vi "String-Based Queued State Machine_ACBMOD.vi"() -> ()   [LabVIEW 2015]
panel:
  in  "OK":bool
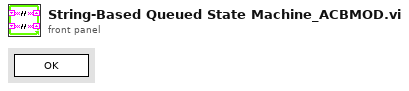
[diagram p1: front panel]
types:
  T1 = enum32{"Invalid", "Standard", "Closed", "Hidden", "Minimized", "Maximized"}
  T2 = enum32{"invalid app kind", "Development System", "Run Time System", "Student Edition", "Embedded LabVIEW", "Evaluation", "Custom"}
  T3 = cluster{"Core":cluster{"Current VI Reference":refnum<vi>, "Close Panel on Exit?":bool}, "Your Boolean data":bool, "Your string data":string}
  T4 = cluster{"Current VI Reference":refnum<vi>, "Close Panel on Exit?":bool}
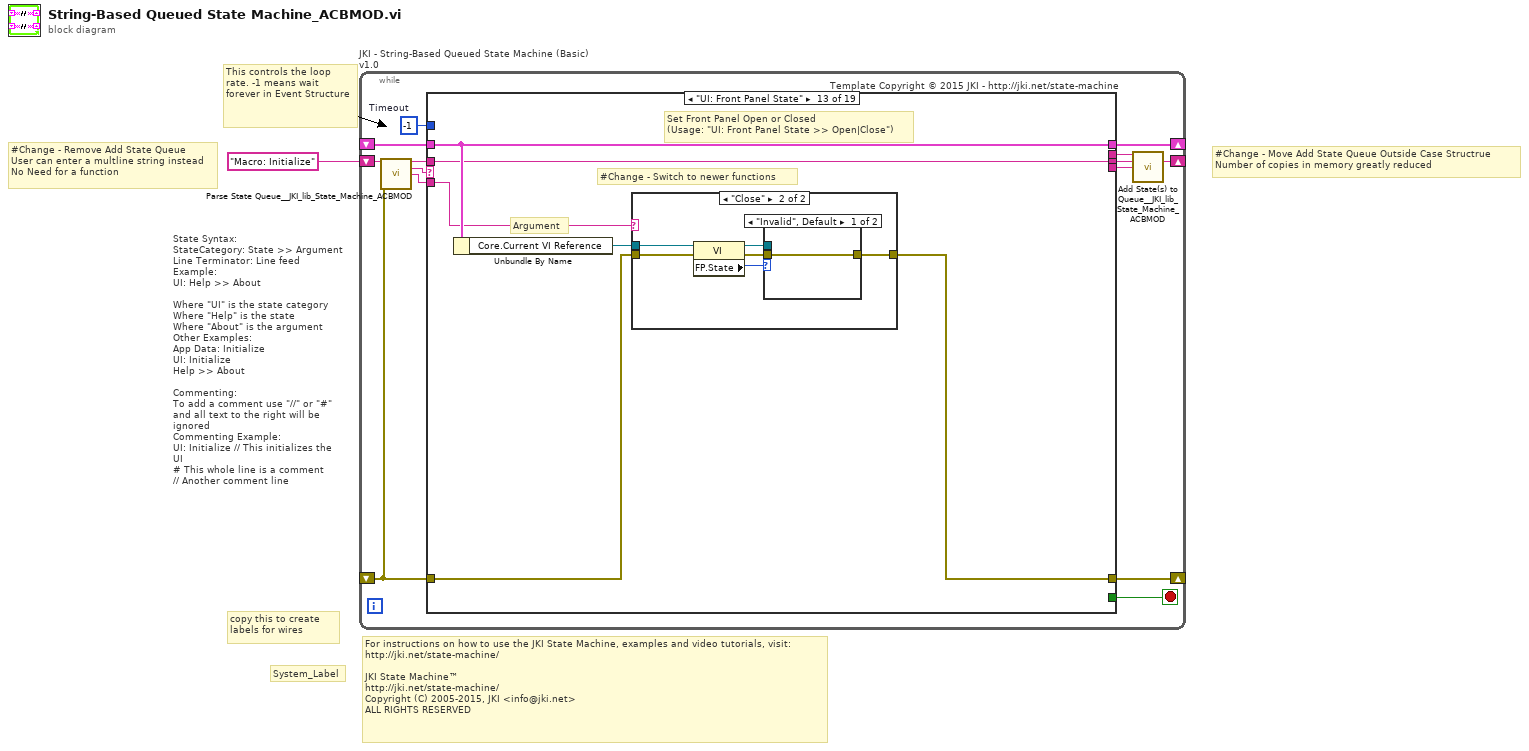
[diagram p0: block diagram]
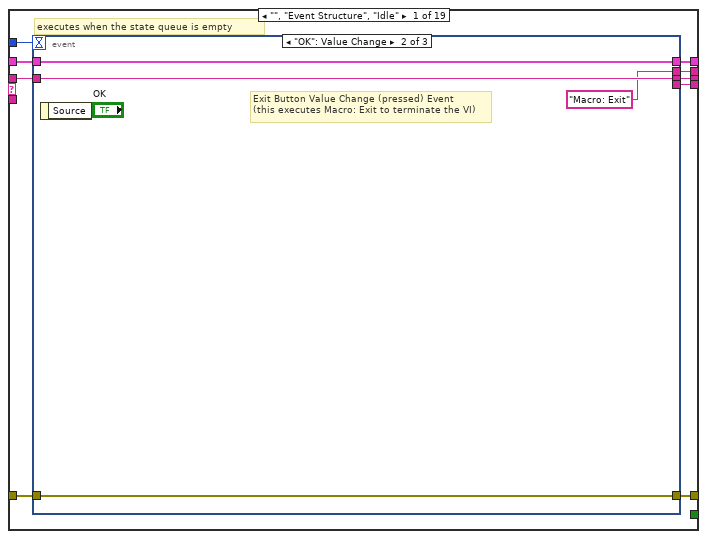
[diagram p2: hidden frame]
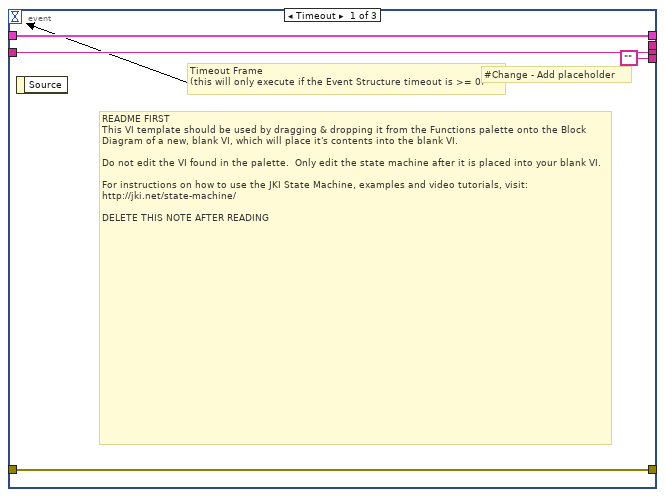
[diagram p3: hidden frame]
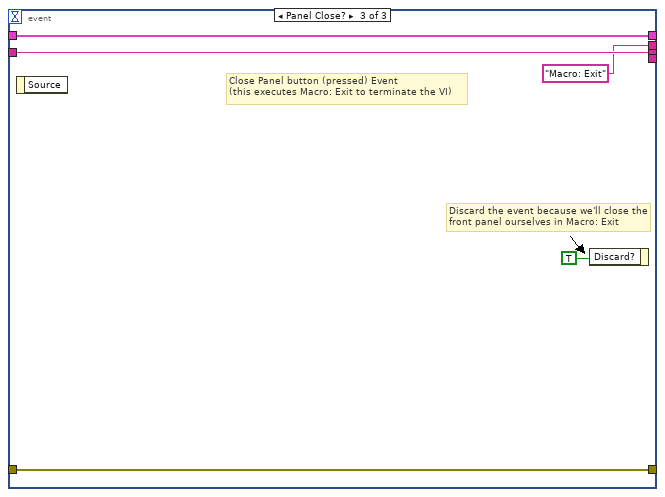
[diagram p4: hidden frame]
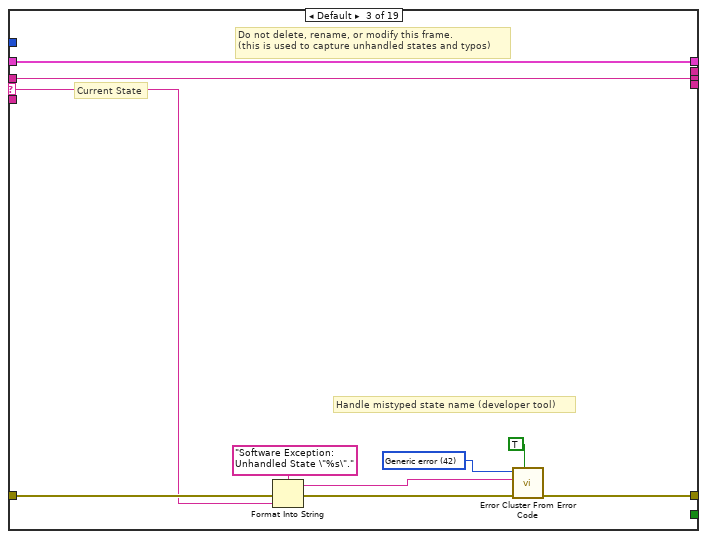
[diagram p6: hidden frame]
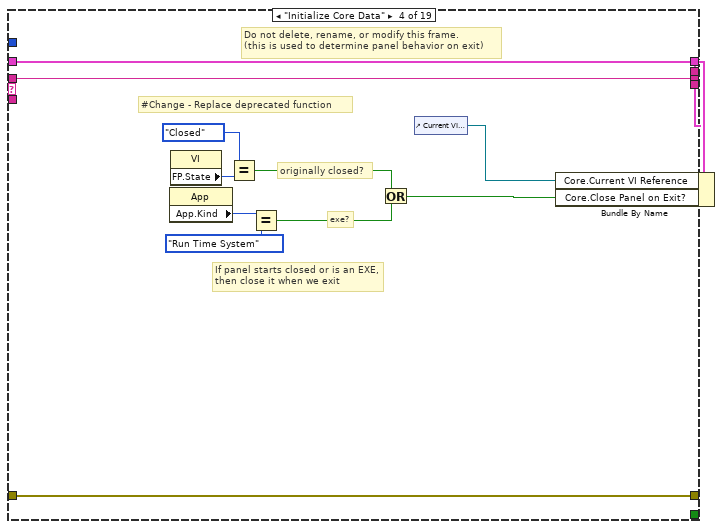
[diagram p7: hidden frame]
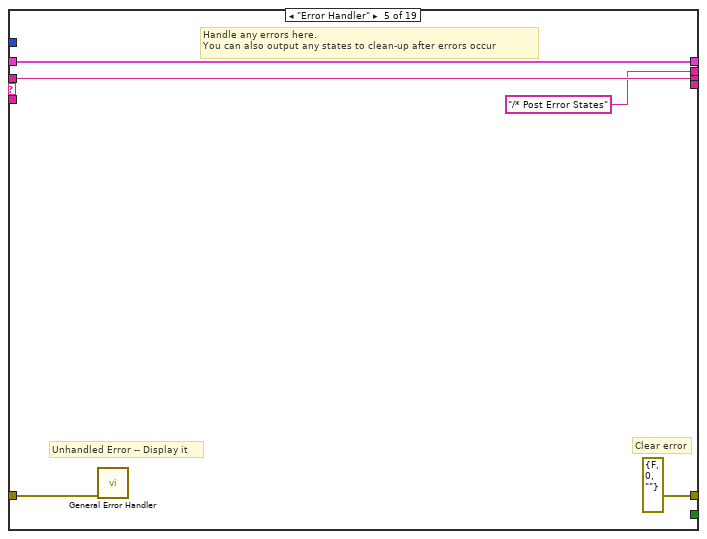
[diagram p8: hidden frame]
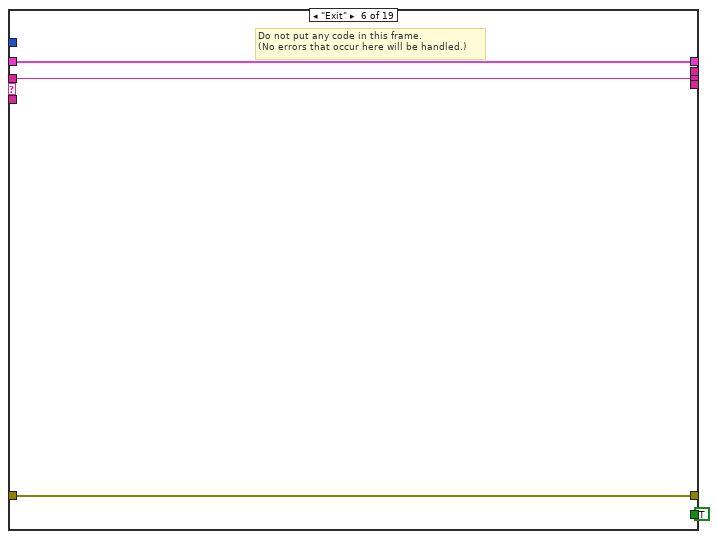
[diagram p9: hidden frame]
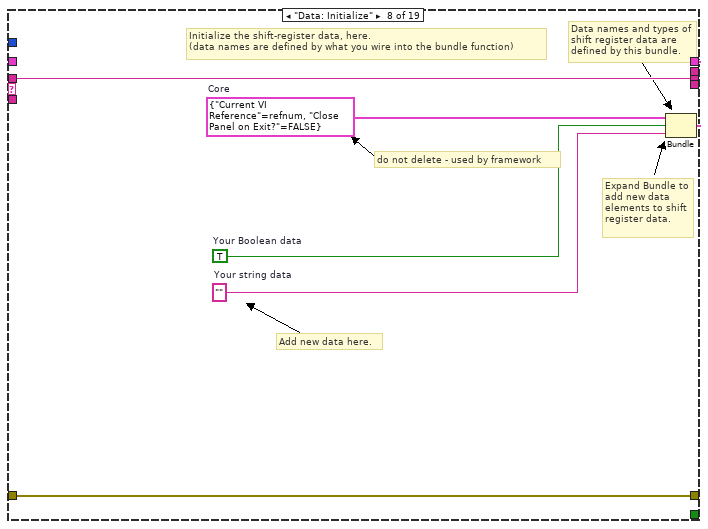
[diagram p11: hidden frame]
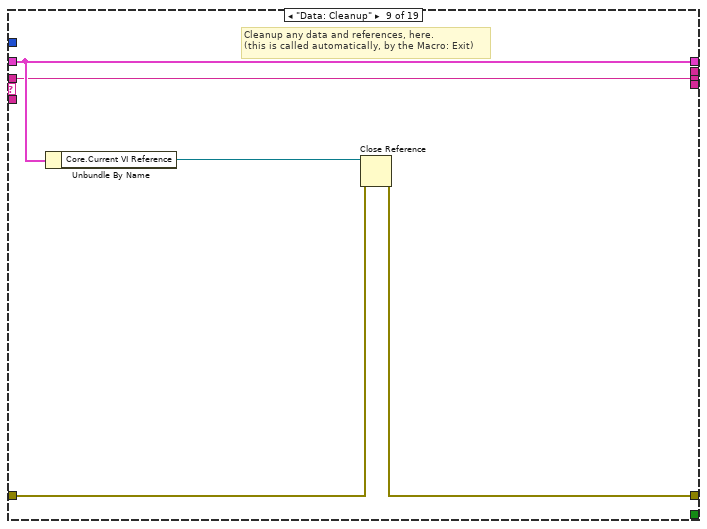
[diagram p12: hidden frame]
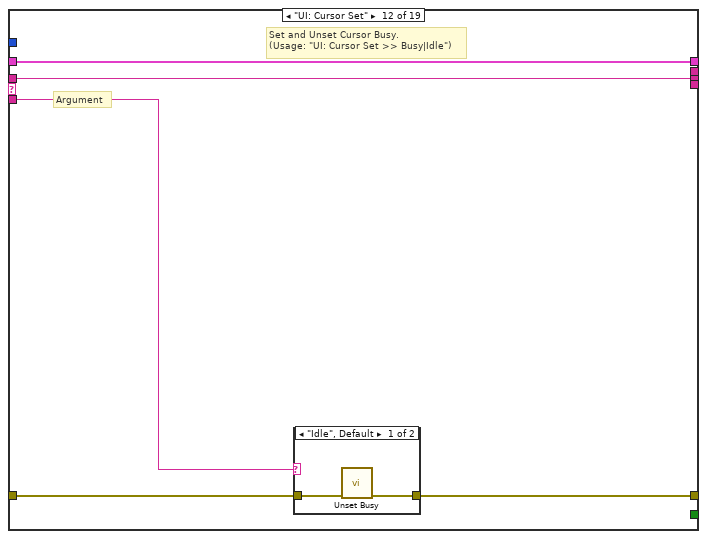
[diagram p15: hidden frame]
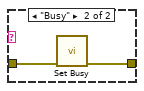
[diagram p16: hidden frame]
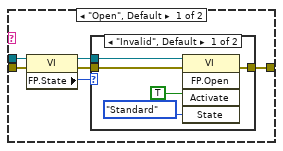
[diagram p17: hidden frame]
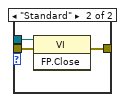
[diagram p19: hidden frame]
diagram:
  # "#Change - Move Add State Queue Outside Case Structrue\nNumber of copies in memory greatly reduced"
  # "#Change - Remove Add State Queue\nUser can enter a multline string instead\nNo Need for a function"
  # "For instructions on how to use the JKI State Machine, examples and video tutorials, visit:\nhttp://jki.net/state-machine/\n\nJKI State Machine™\nhttp://jki.net/state-machine/\nCopyright (C) 2005-2015, JKI <info@jki.net>\nALL RIGHTS RESERVED"
  # "State Syntax:\nStateCategory: State >> Argument\nLine Terminator: Line feed\nExample:\nUI: Help >> About\n\nWhere \"UI\" is the state category\nWhere \"Help\" is the state\nWhere \"About\" is the argument\nOther Examples:\nApp Data: Initialize\nUI: Initialize\nHelp >> About\n\nCommenting:\nTo add a comment use \"//\" or \"#\" and all text to the right will be ignored\nCommenting Example:\nUI: Initialize // This initializes the UI\n# This whole line is a comment\n// Another comment line"
  # "copy this to create labels for wires"
  # "This controls the loop rate. -1 means wait forever in Event Structure"
  # "System_Label"
  n1 = while "JKI - String-Based Queued State Machine (Basic) v1.0" {
    shift-right: [w9] -> _
    shift-left: _ -> [w8]
    shift-right: [w11] -> _
    shift-left: _ -> [w6]
    shift-right: [w4] -> _
    shift-left: "Macro: Initialize" -> [w12]
    stop <- w10 stop-if-true
    w7 = -1  # Timeout
    # "Template Copyright © 2015 JKI - http://jki.net/state-machine"
    n2 = call "Parse State Queue__JKI_lib_State_Machine_ACBMOD.vi"("State Queue"=w12, "Error In"=w6) -> ("Remaining States"=w14:string, "Current State"=w15:string, "Arguments"=w13:string)  [unwired: 11 in]
    n3 = case shown="\"UI: Front Panel State\"" w15 {
      selector: w15 -> [_ _ w42 _ _ _ _ _ _ _ _ _ _ _ _ _ _ _ _]
      tunnel: w14 -> [w24 w38 w41 w51 w64 w68 w72 w75 w81 w86 w89 w92 w101 w129 w133 w137 w145 w148 w151]
      tunnel: w13 -> [_ _ _ _ _ _ _ _ _ _ _ w93 w102 _ _ _ _ _ _]
      tunnel: w8 -> [w22 w39 w44 w58 w66 w71 w73 _ w82 w87 w91 w96 w104 w130 w134 w143 w146 w149 w152]
      tunnel: [w21 w40 w46 w61 errorcluster {"status"=FALSE, "code"=0, "source"=""} ("error out") w70 w74 w79 w83 w88 w90 w94 w105 w131 w135 w144 w147 w150 w153] -> w11
      tunnel: w6 -> [w20 w40 w45 w61 w65 w70 w74 w79 w84 w88 w90 w95 w106 w131 w135 w144 w147 w150 w153]
      tunnel: [w23 w38 w41 w51 w64 w68 w72 w75 w81 w86 w89 w92 w101 w129 w133 w137 w145 w148 w151] -> w5
      tunnel: [_ _ _ _ _ TRUE _ _ _ _ _ _ _ _ _ _ _ _ _] -> w10
      tunnel: [w19 w39 w44 w62 w66 w71 w73 w80 w82 w87 w91 w96 w104 w130 w134 w143 w146 w149 w152] -> w9
      tunnel: w7 -> [w18 _ _ _ _ _ _ _ _ _ _ _ _ _ _ _ _ _ _]
      tunnel: [w17 _ _ _ "/* Post Error States" _ _ _ _ _ _ _ _ _ w132 w136 _ _ _] -> w3
      tunnel: [w16 _ _ _ _ _ _ _ _ _ _ _ _ _ _ _ _ _ _] -> w2
      frame "", "Event Structure", "Idle" {
        # "executes when the state queue is empty"
        n4 = event shown="[1] \"OK\": Value Change" {
          selector: _ -> [_ _ _]
          dyn-events: _ -> [_ _ _]
          timeout: w18 -> [_ _ _]
          tunnel: w24 -> [w26 w30 w34]
          tunnel: [w26 w30 w34] -> w23
          tunnel: w22 -> [w27 w31 w36]
          tunnel: [w28 w32 w37] -> w21
          tunnel: w20 -> [w28 w32 w37]
          tunnel: [w27 w31 w36] -> w19
          tunnel: [_ "Macro: Exit" "Macro: Exit"] -> w17
          tunnel: ["" _ _] -> w16
          event Timeout {
            # "#Change - Add placeholder"
            # "README FIRST\nThis VI template should be used by dragging & dropping it from the Functions palette onto the Block Diagram of a new, blank VI, which will place it's contents into the blank VI.\n\nDo not edit the VI found in the palette.  Only edit the state machine after it is placed into your blank VI.\n\nFor instructions on how to use the JKI State Machine, examples and video tutorials, visit:\nhttp://jki.net/state-machine/\n\nDELETE THIS NOTE AFTER READING"
            # "Timeout Frame\n(this will only execute if the Event Structure timeout is >= 0)"
            n5 = event-data() -> ()  [unwired: 1 in, 1 out]
          }
          event "OK": Value Change {
            # "Exit Button Value Change (pressed) Event\n(this executes Macro: Exit to terminate the VI)"
            n6 = event-data() -> ()  [unwired: 1 in, 1 out]
          }
          event Panel Close? {
            # "Discard the event because we'll close the front panel ourselves in Macro: Exit"
            # "Close Panel button (pressed) Event\n(this executes Macro: Exit to terminate the VI)"
            n7 = event-data() -> ()  [unwired: 1 in, 1 out]
            n8 = event-data("Discard?"=TRUE) -> ()  [unwired: 1 in, 1 out]
          }
        }
      }
      frame "---------- Core ----------" {
        # "Do not put any code in this frame.\n(it is a separator no-op)"
      }
      frame Default {
        w49 = 42 items=["No error", "Argument error", "Memory is full", "Out of zone", "End of file", "File already open", "Generic file I/O error", "File not found", "File permission error", "Disk is full", "Duplicate path", "Too many files open", "System feature not enabled", "Resource file not found", "Cannot add resource", "Resource not found", "Image not found", "Image memory error", "Pen does not exist", "Config type invalid", "Config token not found", "Config parse error", "Config memory error", "Bad external code format", "Bad external code offset", "External code not present", "Null window", "Destroy window error", "Null menu", "Print aborted", "Bad print record", "Print driver error", "Windows error during printing", "Memory error during printing", "Print dialog error", "Generic print error", "Invalid device refnum", "Device not found", "Device parameter error", "Device unit error", "Cannot open device", "Device call aborted", "Generic error", "Cancelled by user", "Object ID too low", "Object ID too high", "Object not in heap", "Unknown heap", "Unknown object (invalid DefProc)", "Unknown object (DefProc not in table)", "Message out of range", "Invalid (null) method", "Unknown message", "Manager call not supported", "Bad address", "Network operation in progress", "Network operation timed out", "Connection is busy", "Network attribute not supported", "Network error", "Address in use", "System out of memory", "Connection aborted", "Connection refused", "Not connected", "Already connected", "Connection closed", "Initialization error (interapplication manager)", "Bad occurrence", "Wait on unbound occurrence handler", "Occurrence queue overflow", "Datalog type conflict", "Unused", "Unrecognized type (interapplication manager)", "Memory corrupt", "Failed to make temporary DLL", "Old CIN version", "Drag socket not found", "Failed to load drop-object", "Failed to register OLE object", "Failed to release OLE object", "Format specifier type mismatch", "Unknown format specifier", "Too few format specifiers", "Too many format specifiers", "Scan failed", "Newer CIN version", "Error converting to variant", "Runtime menu error", "Password tampered", "Variant attribute not found", "Incompatible variant data type", "Event data is not available", "Event Store is not present", "Occurrence is not found", "Event Queue is not created", "Event info is not available", "Refnum passed is NULL", "Error retrieving Class GUID", "Error retrieving CoClass GUID", "Error retrieving TypeLib GUID.", "Bad built application magic bytes.", "Specific driver is different from the specific driver associated with the Logical Name.", "There is no session opened to the class driver.", "Max Error", "MAX - Error with config objects", "MAX - Error loading configuration", "MAX - Group not supported"]
        # "Current State"
        # "Do not delete, rename, or modify this frame.\n(this is used to capture unhandled states and typos)"
        # "Handle mistyped state name (developer tool)"
        n9 = Format Into String(format string="Software Exception: Unhandled State \"%s\"." ("message"), error in=w45, w42) -> (resulting string=w48:string, error out=w47:errorcluster)  [unwired: 1 in]
        n10 = call <vilib>:"Error Cluster From Error Code.vi"("show call chain? (False)"=TRUE, "error in (no error)"=w47, "error message (\"\")"=w48, "error code (0)"=w49) -> ("error out"=w46:errorcluster)  [unwired: 5 in]
      }
      frame "Initialize Core Data" {
        # "#Change - Replace deprecated function"
        # "Do not delete, rename, or modify this frame.\n(this is used to determine panel behavior on exit)"
        # "originally closed?"
        # "exe?"
        # "If panel starts closed or is an EXE, then close it when we exit"
        n11 = property class="App"() -> ("App.Kind"=w55:T2)  [unwired: 2 in, 2 out]
        n12 = property class="VI"() -> ("FP.State"=w54:T1)  [unwired: 2 in, 2 out]
        n13 = Equal?(x=T1."Closed", y=w54) -> (x = y?=w52:bool)
        n14 = Equal?(x=w55, y=T2."Run Time System" ("Application:Kind")) -> (x = y?=w59:bool)
        n15 = Or(x=w52, y=w59) -> (x .or. y?=w57:bool)
        n16 = control-ref of="Current VI Reference"() -> (w56:refnum<vi>)
        n17 = Bundle By Name(cluster=w58, "Core.Current VI Reference"=w56, "Core.Close Panel on Exit?"=w57) -> (w62:T3)
      }
      frame "Error Handler" {
        # "Unhandled Error -- Display it"
        # "Handle any errors here.\nYou can also output any states to clean-up after errors occur"
        # "Clear error"
        n18 = call <vilib>:"General Error Handler.vi"("error in (no error)"=w65) -> ()  [unwired: 10 in, 5 out]
      }
      frame "Exit" {
        # "Do not put any code in this frame.\n(No errors that occur here will be handled.)"
      }
      frame "---------- Data ----------" {
        # "Do not put any code in this frame.\n(It is a separator no-op. You can make a copy of this frame to create a new Data frame)"
      }
      frame "Data: Initialize" {
        w76 = T4 {"Current VI Reference"=refnum, "Close Panel on Exit?"=FALSE}  # Core
        w78 = TRUE  # Your Boolean data
        w77 = ""  # Your string data
        # "do not delete - used by framework"
        # "Expand Bundle to add new data elements to shift register data."
        # "Add new data here."
        # "Data names and types of shift register data are defined by this bundle."
        # "Initialize the shift-register data, here.\n(data names are defined by what you wire into the bundle function)"
        n19 = Bundle("Core"=w76, "Your Boolean data"=w78, "Your string data"=w77) -> (w80:T3)  [unwired: 1 in]
      }
      frame "Data: Cleanup" {
        # "Cleanup any data and references, here.\n(this is called automatically, by the Macro: Exit)"
        n20 = Unbundle By Name(w82) -> ("Core.Current VI Reference"=w85:refnum<vi>)
        n21 = Close Reference(reference=w85, error in (no error)=w84) -> (error out=w83:errorcluster)
      }
      frame "---------- UI ----------" {
        # "Do not put any code in this frame.\n(It is a separator no-op. You can make a copy of this frame to create a new UI frame)"
      }
      frame "UI: Initialize" {
        # "Initialize the User Interface, here.\n(this is called automatically, by the Macro: Init)"
      }
      frame "UI: Cursor Set" {
        # "Argument"
        # "Set and Unset Cursor Busy.\n(Usage: \"UI: Cursor Set >> Busy|Idle\")"
        n22 = case shown="\"Idle\", Default" w93 {
          tunnel: w95 -> [w98 w100]
          tunnel: [w97 w99] -> w94
          frame "Idle", Default {
            n23 = call <vilib>:"Unset Busy.vi"("error in (no error)"=w98) -> ("error out"=w97:errorcluster)  [unwired: 10 in]
          }
          frame "Busy" {
            n24 = call <vilib>:"Set Busy.vi"("error in (no error)"=w100) -> ("error out"=w99:errorcluster)  [unwired: 9 in, 1 out]
          }
        }
      }
      frame "UI: Front Panel State" {
        # "#Change - Switch to newer functions"
        # "Argument"
        # "Set Front Panel Open or Closed\n(Usage: \"UI: Front Panel State >> Open|Close\")"
        n25 = Unbundle By Name(w104) -> ("Core.Current VI Reference"=w103:refnum<vi>)
        n26 = case shown="\"Close\"" w102 {
          tunnel: w106 -> [w110 w123]
          tunnel: [w112 w124] -> w105
          tunnel: w103 -> [w111 w121]
          frame "Open", Default {
            n27 = property class="VI"(reference=w111, error in=w110) -> (reference out=w108:refnum<vi>, error out=w109:errorcluster, "FP.State"=w107:T1)
            n28 = case shown="\"Invalid\", Default" w107 {
              tunnel: [w115 w118] -> w112
              tunnel: w109 -> [w114 w118]
              tunnel: w108 -> [w113 _]
              frame "Invalid", Default {
                n29 = invoke class="VI" method="FP.Open"(reference=w113, error in=w114, "Activate"=TRUE, "State"=T1."Standard") -> (error out=w115:errorcluster)  [unwired: 1 in, 4 out]
              }
              frame "Standard" {
              }
            }
          }
          frame "Close" {
            n30 = property class="VI"(reference=w121, error in=w123) -> (reference out=w120:refnum<vi>, error out=w122:errorcluster, "FP.State"=w119:T1)
            n31 = case shown="\"Invalid\", Default" w119 {
              tunnel: [w125 w128] -> w124
              tunnel: w122 -> [w125 w127]
              tunnel: w120 -> [_ w126]
              frame "Invalid", Default {
              }
              frame "Standard" {
                n32 = invoke class="VI" method="FP.Close"(reference=w126, error in=w127) -> (error out=w128:errorcluster)  [unwired: 1 in, 2 out]
              }
            }
          }
        }
      }
      frame "---------- Macro ----------" {
        # "Do not put any code in this frame.\n(It is a separator no-op. You can make a copy of this frame to create a new Macro frame)"
      }
      frame "Macro: Initialize" {
        w132 = "Data: Initialize\nInitialize Core Data\nUI: Initialize\nUI: Front Panel State >> Open"  # Data: Initialize Initialize Core Data UI: Initialize UI: Front Panel State >> Open
        # "Initialization Macro\n(This is called once, when the VI starts)"
      }
      frame "Macro: Exit" {
        # "Exit Macro\n(This is called once, when the VI exits)"
        n33 = Unbundle By Name(w143) -> ("Core.Close Panel on Exit?"=w142:bool)
        n34 = Select(t="UI: Front Panel State >> Close", s=w142, f="") -> (s? t:f=w139:string)
        n35 = call "Add State(s) to Queue__JKI_lib_State_Machine_ACBMOD.vi"("State(s) in (\"\")"=w139, "State(s) at Back (\"\")"="Data: Cleanup\nExit") -> ("States Out"=w136:string)  [unwired: 13 in]
      }
      frame "---------- New Category ----------" {
        # "Template Separator\n(You can make a copy of, or modify, this frame)"
      }
      frame "New Category: 1" {
        # "Your code here.\n(You can make a copy of, or modify, this frame)"
      }
      frame "New Category: 2" {
        # "Your code here.\n(You can make a copy of, or modify, this frame)"
      }
    }
    n36 = call "Add State(s) to Queue__JKI_lib_State_Machine_ACBMOD.vi"("State(s) in Front (\"\")"=w3, "State(s) in (\"\")"=w5, "State(s) at Back (\"\")"=w2) -> ("States Out"=w4:string)  [unwired: 12 in]
  }
